vi "HH_ProcData.vi"(4 "isMarker":bool, 6 "Channel":u32, 7 "MHData in":T2, 8 "MH_VisThread_QRef":T1, 9 "dtime":u32, 10 "photon":bool, 11 "truetime":u64) -> (5 "MHData out":T2)   [LabVIEW 2010]
uses:
  Types/HH_VisThread_QData.ctl
  Types/HH_VisThread_QCmds.ctl
  Types/HH_DataProcThread_Data.ctl
  Types/HH_VisThread_QRef.ctl
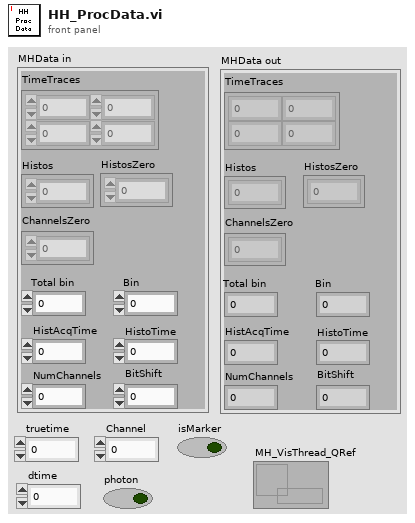
[diagram p1: front panel]
types:
  T1 = typedef "HH_VisThread_QRef.ctl" = refnum<queue>
  T2 = typedef "HH_DataProcThread_Data.ctl" = cluster{"TimeTraces":u32[][], "BitShift":i16, "NumChannels":i32, "Total bin":u64, "Bin":i32, "HistAcqTime":i32, "HistoTime":u64, "Histos":u32[][], "HistosZero":u32[][], "ChannelsZero":u32[]}
  T3 = typedef "HH_VisThread_QData.ctl" = cluster{"Histos":u32[][], "Cmd":T4, "TimeTrace":u32[][], "Bin":i32, "Total bin":u64, "Status":string, "Resol":dbl, "DeltaT":dbl, "nChannels":i32}
  T4 = typedef "HH_VisThread_QCmds.ctl" = enum16{"_none_", "Resol", "nChannels", "DeltaT", "Histo", "TTrace", "Status"}
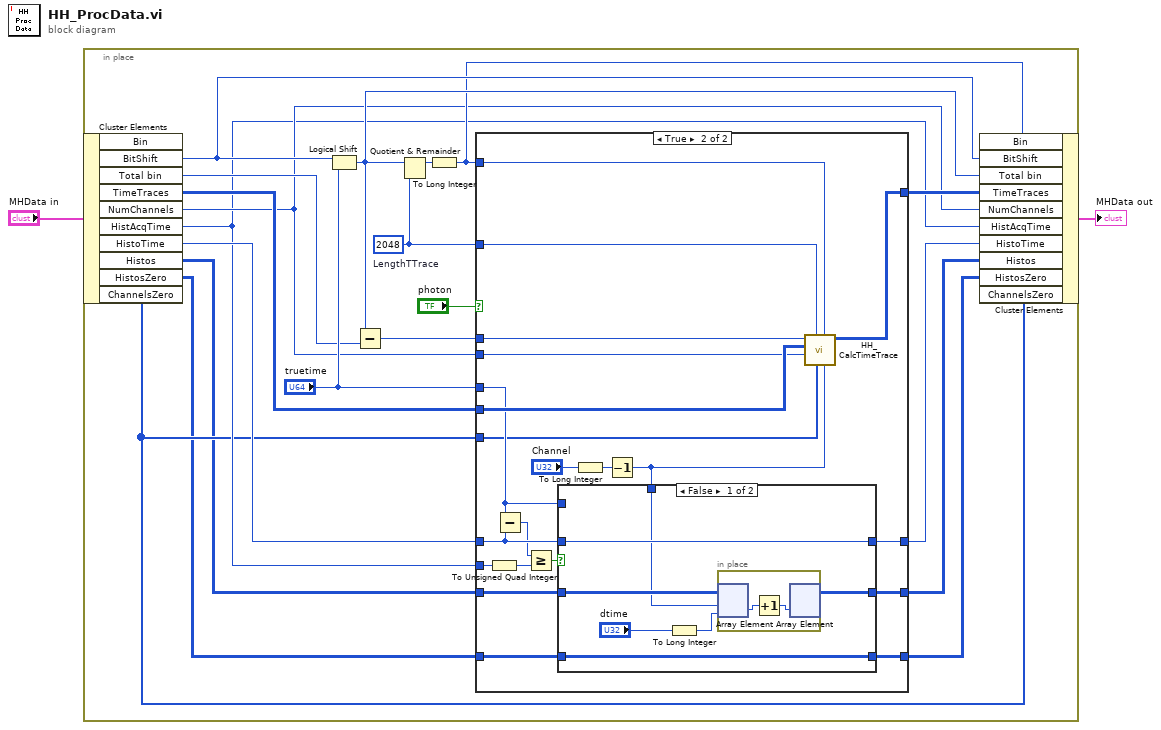
[diagram p0: block diagram]
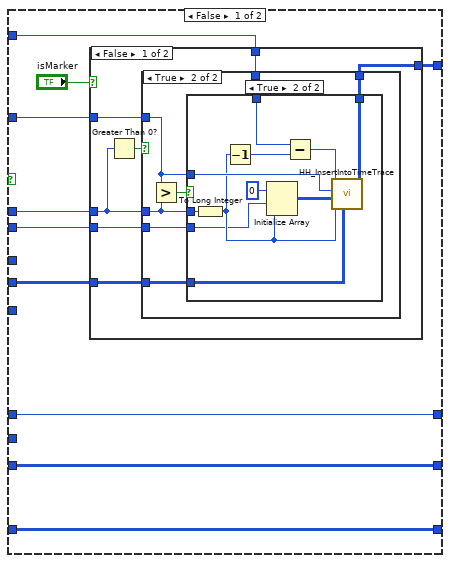
[diagram p2: hidden frame]
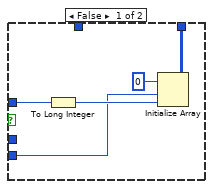
[diagram p4: hidden frame]
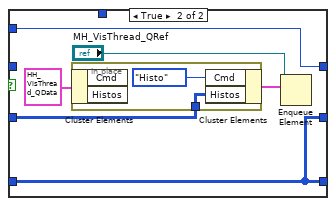
[diagram p6: hidden frame]
diagram:
  n1 = in-place {
    w21 = u64 2048  # LengthTTrace
    n2 = in-place-cluster #1("MHData in") -> ("BitShift"=w12:i16, "Total bin"=w17:u64, "TimeTraces"=w16:u32[][], "NumChannels"=w10:i32, "HistAcqTime"=w8:i32, "HistoTime"=w15:u64, "Histos"=w4:u32[][], "HistosZero"=w6:u32[][], "ChannelsZero"=w7:u32[])  [unwired: 1 out]
    n3 = Logical Shift(y=w12, x="truetime") -> (x << y=w13:u64)
    n4 = Subtract(x=w13, y=w17) -> (x-y=w19:u64)
    n5 = Quotient & Remainder(x=w13, y=w21) -> (x-y*floor(x/y)=w20:u64)  [unwired: 1 out]
    n6 = To Long Integer(number=w20) -> (32bit integer=w11:i32)
    n7 = case shown="True" "photon" {
      tunnel: [w32 w82] -> w14
      tunnel: w4 -> [w23 w85]
      tunnel: [w23 w84] -> w3
      tunnel: w11 -> [w31 w81]
      tunnel: w21 -> [w30 w83]
      tunnel: w16 -> [w29 w80]
      tunnel: w10 -> [w28 w74]
      tunnel: w19 -> [w27 w79]
      tunnel: "truetime" -> [_ w76]
      tunnel: w8 -> [_ w77]
      tunnel: w15 -> [w25 w75]
      tunnel: [w25 w78] -> w9
      tunnel: w6 -> [w24 w73]
      tunnel: [w24 w65] -> w5
      tunnel: w7 -> [_ w68]
      frame False {
        n8 = case shown="False" "isMarker" {
          tunnel: [w38 w64] -> w32
          tunnel: w31 -> [w37 _]
          tunnel: w30 -> [w36 _]
          tunnel: w29 -> [w35 w64]
          tunnel: w28 -> [w34 _]
          tunnel: w27 -> [w33 _]
          frame False {
            n9 = Greater Than 0?(x=w33) -> (x > 0?=w39:bool)
            n10 = case shown="True" w39 {
              tunnel: [w40 w43] -> w38
              tunnel: w36 -> [_ w44]
              tunnel: w33 -> [_ w46]
              tunnel: w37 -> [_ w45]
              tunnel: w35 -> [w40 w41]
              tunnel: w34 -> [_ w42]
              frame False {
              }
              frame True {
                n11 = Greater?(x=w44, y=w46) -> (0:w47:bool)
                n12 = case shown="True" w47 {
                  tunnel: w46 -> [_ w63]
                  tunnel: w45 -> [_ w62]
                  tunnel: [w50 w60] -> w43
                  tunnel: w44 -> [w51 w56]
                  tunnel: w42 -> [w48 w53]
                  tunnel: w41 -> [_ w55]
                  frame False {
                    n13 = To Long Integer(number=w51) -> (32bit integer=w49:i32)
                    n14 = Initialize Array(u32 0 ("element"), w48, w49) -> (w50:u32[][])
                  }
                  frame True {
                    n15 = To Long Integer(number=w63) -> (32bit integer=w54:i32)
                    n16 = Decrement(x=w54) -> (x-1=w58:i32)
                    n17 = Initialize Array(u32 0 ("element"), w53, w54) -> (w61:u32[][])
                    n18 = Subtract(x=w62, y=w58) -> (x-y=w57:i32)
                    n19 = call "HH_InsertIntoTimeTrace.vi"("TimeTrace in"=w55, "NumVals"=w54, "Vals"=w61, "LengthTTrace"=w56, "TimeTraceBin"=w57) -> ("TimeTrace out"=w60:u32[][])  [unwired: 6 in]
                  }
                }
              }
            }
          }
          frame True {
          }
        }
      }
      frame True {
        n20 = To Unsigned Quad Integer(1:w77) -> (0:w71:u64)
        n21 = Subtract(x=w76, y=w75) -> (x-y=w67:u64)
        n22 = Greater Or Equal?(x=w67, y=w71) -> (x >= y?=w72:bool)
        n23 = To Long Integer(number="Channel") -> (32bit integer=w70:i32)
        n24 = Decrement(x=w70) -> (x-1=w69:i32)
        n25 = case shown="False" w72 {
          tunnel: w85 -> [w92 w99]
          tunnel: [w90 w95] -> w84
          tunnel: w69 -> [w87 _]
          tunnel: w75 -> [w91 _]
          tunnel: [w91 w100] -> w78
          tunnel: w76 -> [_ w100]
          tunnel: w73 -> [w86 w95]
          tunnel: [w86 w95] -> w65
          frame False {
            n26 = To Long Integer(number="dtime") -> (32bit integer=w88:i32)
            n27 = in-place {
              n28 = in-place-array #2(w92, w87, w88) -> (w94:u32)
              n29 = Increment(x=w94) -> (x+1=w93:u32)
              n30 = in-place-array #2(w93) -> (w90:u32[][])  [unwired: 2 out]
            }
          }
          frame True {
            n31 = in-place {
              in-place-border: w99 -> [w101]
              n32 = in-place-cluster #3(T3 {"Histos"=[], "Cmd"=enum."_none_", "TimeTrace"=[], "Bin"=0, "Total bin"=0, "Status"="", "Resol"=0.0, "DeltaT"=0.0, "nChannels"=0} ("element")) -> ()  [unwired: 2 out]
              n33 = in-place-cluster #3("Cmd"=HH_VisThread_QCmds."Histo", "Histos"=w101) -> (w98:T3)
            }
            n34 = Enqueue Element(queue="MH_VisThread_QRef", element=w98) -> ()  [unwired: 2 in, 3 out]
          }
        }
        n35 = call "HH_CalcTimeTrace.vi"("Channel"=w69, "Bin"=w81, "ChannelsZero"=w68, "LengthTTrace"=w83, "NumChannels"=w74, "TimeTraces in"=w80, "DeltaTotalBin"=w79) -> ("TimeTraces out"=w82:u32[][])  [unwired: 4 in]
      }
    }
    n36 = in-place-cluster #1("Bin"=w11, "BitShift"=w12, "Total bin"=w13, "TimeTraces"=w14, "NumChannels"=w10, "HistAcqTime"=w8, "HistoTime"=w9, "Histos"=w3, "HistosZero"=w5, "ChannelsZero"=w7) -> (→"MHData out":T2)
  }
